vi "CoomwithHVS.vi"() -> ()   [LabVIEW 2013]
panel:
  in  "stop":bool
  out "return count":u32
  out "Bytes at port":u32
  out "read buffer":string
  in  "port":refnum<visa-resource-name>
  in  "error in (no error)":errorcluster
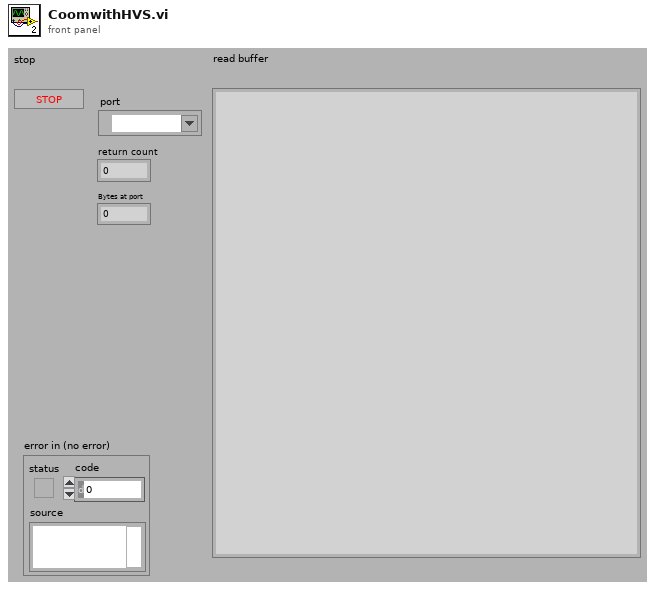
[diagram p1: front panel]
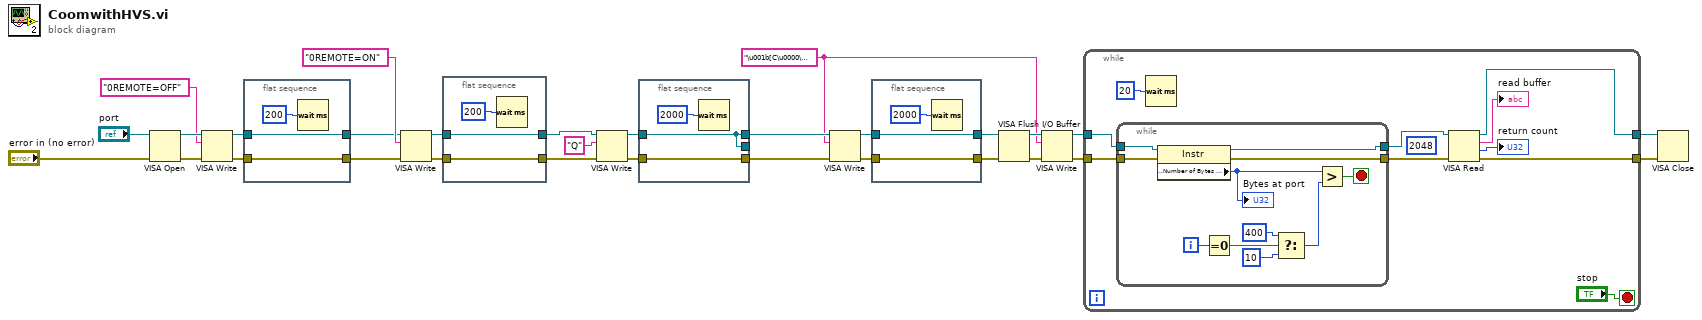
[diagram p0: block diagram]
diagram:
  w3 = "\u001b[C\u0000\u0000" ("write buffer")
  n1 = VISA Open(error in (no error)="error in (no error)", VISA resource name="port") -> (VISA resource name=w25:refnum<visa-resource-name>, error out=w26:errorcluster)  [unwired: 3 in]
  n2 = VISA Write(VISA resource name=w25, write buffer="0REMOTE=OFF", error in (no error)=w26) -> (VISA resource name out=w19:refnum<visa-resource-name>, error out=w21:errorcluster)  [unwired: 1 out]
  n3 = flat-sequence {
    tunnel: w21 -> [w32]
    tunnel: [w32] -> w20
    tunnel: w19 -> [w31]
    tunnel: [w31] -> w18
    frame #0 {
      n4 = Wait (ms)(milliseconds to wait=u32 200) -> ()  [unwired: 1 out]
    }
  }
  n5 = VISA Write(VISA resource name=w18, write buffer="0REMOTE=ON", error in (no error)=w20) -> (VISA resource name out=w15:refnum<visa-resource-name>, error out=w17:errorcluster)  [unwired: 1 out]
  n6 = flat-sequence {
    tunnel: w17 -> [w35]
    tunnel: [w35] -> w16
    tunnel: w15 -> [w34]
    tunnel: [w34] -> w14
    frame #0 {
      n7 = Wait (ms)(milliseconds to wait=u32 200) -> ()  [unwired: 1 out]
    }
  }
  n8 = VISA Write(VISA resource name=w14, write buffer="Q", error in (no error)=w16) -> (VISA resource name out=w12:refnum<visa-resource-name>, error out=w13:errorcluster)  [unwired: 1 out]
  n9 = flat-sequence {
    tunnel: w13 -> [w38]
    tunnel: [w38] -> w10
    tunnel: w12 -> [w37]
    tunnel: [w37] -> _
    tunnel: [w37] -> w11
    frame #0 {
      n10 = Wait (ms)(milliseconds to wait=u32 2000) -> ()  [unwired: 1 out]
    }
  }
  n11 = VISA Write(VISA resource name=w11, write buffer=w3, error in (no error)=w10) -> (VISA resource name out=w8:refnum<visa-resource-name>, error out=w9:errorcluster)  [unwired: 1 out]
  n12 = flat-sequence {
    tunnel: w9 -> [w41]
    tunnel: [w41] -> w6
    tunnel: w8 -> [w40]
    tunnel: [w40] -> w7
    frame #0 {
      n13 = Wait (ms)(milliseconds to wait=u32 2000) -> ()  [unwired: 1 out]
    }
  }
  n14 = VISA Flush I/O Buffer(VISA resource name=w7, error in (no error)=w6) -> (VISA resource name out=w5:refnum<visa-resource-name>, error out=w4:errorcluster)  [unwired: 1 in]
  n15 = VISA Write(VISA resource name=w5, write buffer=w3, error in (no error)=w4) -> (VISA resource name out=w2:refnum<visa-resource-name>, error out=w1:errorcluster)  [unwired: 1 out]
  n16 = while {
    tunnel: [w52] -> w28
    tunnel: [w51] -> w27
    tunnel: w2 -> [w45]
    tunnel: w1 -> [w44]
    stop <- "stop" stop-if-true
    (unwired) u32 2048 ("byte count")
    n17 = while {
      tunnel: [w63] -> w50
      tunnel: w45 -> [w60]
      tunnel: w44 -> [w59]
      tunnel: [w58] -> w43
      i -> [w57]
      stop <- w61 stop-if-true
      n18 = property class="Instr"(reference=w60, error in=w59) -> (reference out=w63:refnum<visa-resource-name>, error out=w58:errorcluster, "Serial Settings:Number of Bytes at Serial Port"=w62:u32)
      "Bytes at port" <- w62
      n19 = Equal To 0?(x=w57) -> (x = 0?=w56:bool)
      n20 = Select(t=u32 400 ("y"), s=w56, f=u32 10 ("y")) -> (s? t:f=w53:u32)
      n21 = Greater?(x=w62, y=w53) -> (0:w61:bool)
    }
    n22 = Wait (ms)(milliseconds to wait=u32 20) -> ()  [unwired: 1 out]
    n23 = VISA Read(VISA resource name=w50, error in (no error)=w43) -> (VISA resource name out=w52:refnum<visa-resource-name>, read buffer=→"read buffer":string, return count=→"return count":u32, error out=w51:errorcluster)  [unwired: 1 in]
  }
  n24 = VISA Close(VISA resource name=w28, error in (no error)=w27) -> ()  [unwired: 1 out]
